vi "XY Increment move.vi"(4 "- Y":bool, 5 "- X":bool, 6 "+ Y":bool, 7 "+ X":bool, 8 "error in (no error)":errorcluster, 11 "Motion in":refnum<class "Motion.lvclass">=refnum) -> (0 "error out":errorcluster, 3 "Motion out":refnum<class "Motion.lvclass">)   [LabVIEW 2016, in "Motion.lvclass"]
uses:
  Motion.lvclass
  A3200 Folder/A3200.lvclass
panel:
  in  "Distance":dbl[](array[numeric])=[0.01] format="%#_13g"
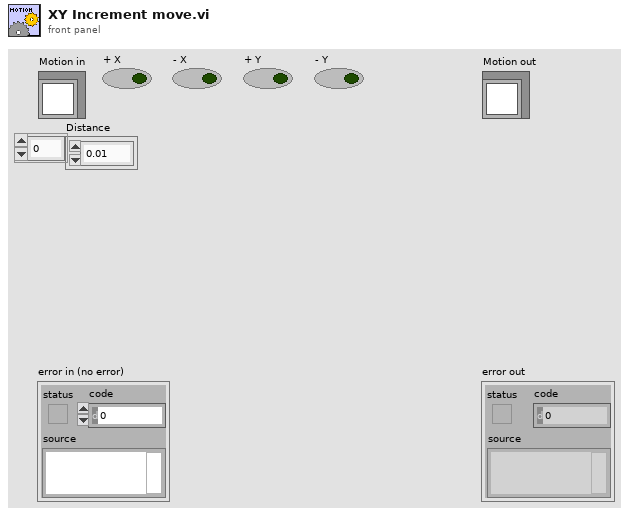
[diagram p1: front panel]
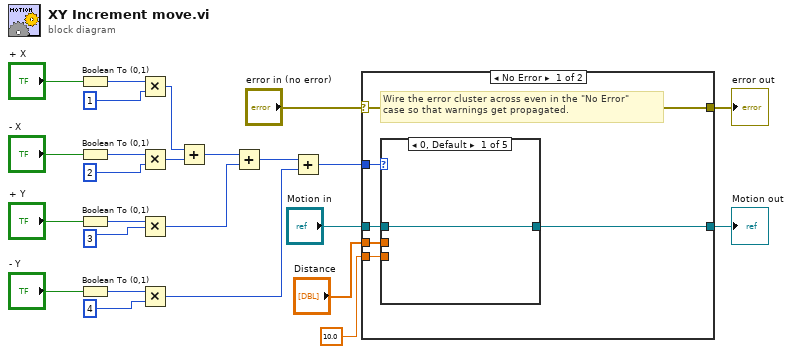
[diagram p0: block diagram]
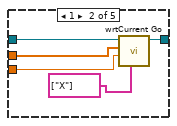
[diagram p2: hidden frame]
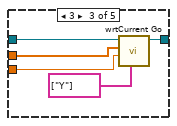
[diagram p3: hidden frame]
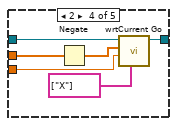
[diagram p4: hidden frame]
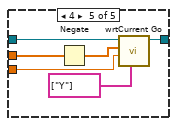
[diagram p5: hidden frame]
diagram:
  n1 = Boolean To (0,1)(Boolean="+ X") -> (0, 1=w18:i16)
  n2 = Boolean To (0,1)(Boolean="- X") -> (0, 1=w15:i16)
  n3 = Boolean To (0,1)(Boolean="+ Y") -> (0, 1=w12:i16)
  n4 = Boolean To (0,1)(Boolean="- Y") -> (0, 1=w9:i16)
  n5 = Multiply(x=w18, y=i16 1) -> (x*y=w7:i16)
  n6 = Multiply(x=w15, y=i16 2) -> (x*y=w6:i16)
  n7 = Multiply(x=w12, y=i16 3) -> (x*y=w4:i16)
  n8 = Multiply(x=w9, y=i16 4) -> (x*y=w2:i16)
  n9 = Add(x=w7, y=w6) -> (x+y=w5:i16)
  n10 = Add(x=w5, y=w4) -> (x+y=w3:i16)
  n11 = Add(x=w3, y=w2) -> (x+y=w1:i16)
  n12 = case shown="No Error" "error in (no error)" {
    selector: "error in (no error)" -> [w31 w56]
    tunnel: [w31 w56] -> w24
    tunnel: [w29 w55] -> w22
    tunnel: "Motion in" -> [w30 w55]
    tunnel: "Distance" -> [w26 _]
    tunnel: 10.0 ("Speed") -> [w27 _]
    tunnel: w1 -> [w28 _]
    frame No Error {
      # "Wire the error cluster across even in the \"No Error\"\ncase so that warnings get propagated."
      n13 = case shown="0, Default" w28 {
        tunnel: w30 -> [w32 w37 w42 w48 w54]
        tunnel: [w32 w36 w41 w47 w53] -> w29
        tunnel: w27 -> [_ w35 w40 w46 w52]
        tunnel: w26 -> [_ w34 w39 w43 w49]
        frame 0, Default {
        }
        frame 1 {
          n14 = call-dynamic "wrtCurrent Go.vi"("Axis"=string[] ["X"], "Speed"=w35, "Distance"=w34, "Motion in"=w37) -> ("Motion out"=w36:refnum<class "Motion.lvclass">)  [unwired: 6 in, 1 out]
        }
        frame 3 {
          n15 = call-dynamic "wrtCurrent Go.vi"("Axis"=string[] ["Y"], "Speed"=w40, "Distance"=w39, "Motion in"=w42) -> ("Motion out"=w41:refnum<class "Motion.lvclass">)  [unwired: 6 in, 1 out]
        }
        frame 2 {
          n16 = Negate(x=w43) -> (-x=w44:dbl[])
          n17 = call-dynamic "wrtCurrent Go.vi"("Axis"=string[] ["X"], "Speed"=w46, "Distance"=w44, "Motion in"=w48) -> ("Motion out"=w47:refnum<class "Motion.lvclass">)  [unwired: 6 in, 1 out]
        }
        frame 4 {
          n18 = Negate(x=w49) -> (-x=w50:dbl[])
          n19 = call-dynamic "wrtCurrent Go.vi"("Axis"=string[] ["Y"], "Speed"=w52, "Distance"=w50, "Motion in"=w54) -> ("Motion out"=w53:refnum<class "Motion.lvclass">)  [unwired: 6 in, 1 out]
        }
      }
    }
    frame Error {
    }
  }
  "error out" <- w24
  "Motion out" <- w22
